vi "errorCheckArrayIndex.vi"(9 "<single path ele>":string, 10 "<req. obj>":string, 11 "Variant":variant) -> (3 "value":string)   [LabVIEW 2015, in "Zen Analytics.lvclass"]
uses:
  Zen Analytics.lvclass
  <vilib>/Utility/Data Type/Type Definitions/Data Type.ctl
  <vilib>/regexp/Match Regular Expression.xnode
  <vilib>/Utility/Data Type/NI_Data Type.lvlib
panel:
  out "error out":errorcluster
  in  "error in (no error)":errorcluster
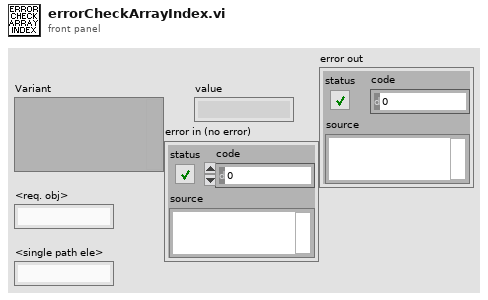
[diagram p1: front panel]
types:
  T1 = typedef "NI_Data Type.lvlib/Data Type.ctl" = enum8{"Invalid Type", "Void", "I8", "I16", "I32", "I64", "U8", "U16", "U32", "U64", "Single Float", "Double Float", "Extended Float", "Single Complex", "Double Complex", "Extended Complex", "Enum U8", "Enum U16", "Enum U32", "Enum U64", "Single Float With Unit", "Double Float With Unit", "Extended Float With Unit", "Single Complex with Unit", "Double Complex with Unit", "Extended Complex with Unit", "Boolean", "String", "Path", "Picture", "Tag", "Array", "Cluster", "Variant", "LV Variant", "Waveform", "Timestamp", "Digital Waveform", "Digital Data", "ExpressData", "Refnum", "External Data", "VI", "Poly VI", "LabVIEW Class Instance", "Fixed Point"}
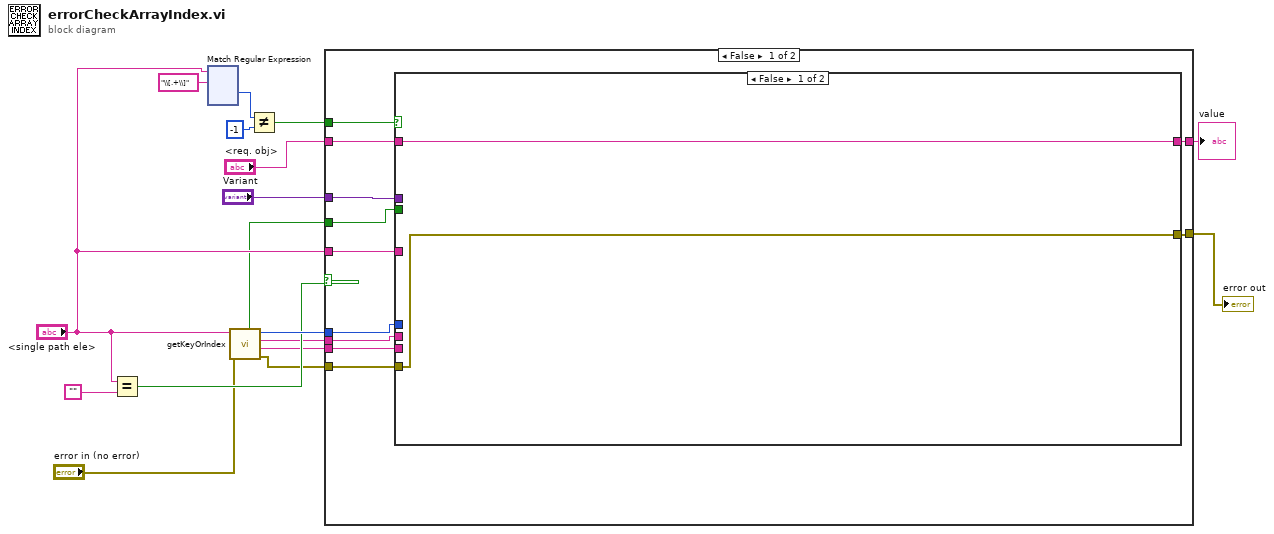
[diagram p0: block diagram]
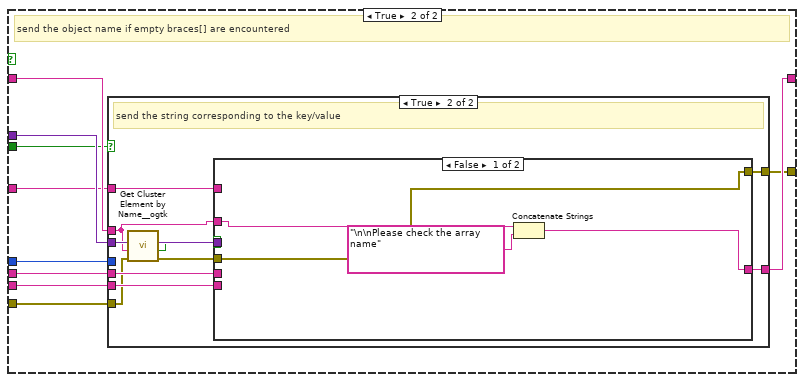
[diagram p2: hidden frame]
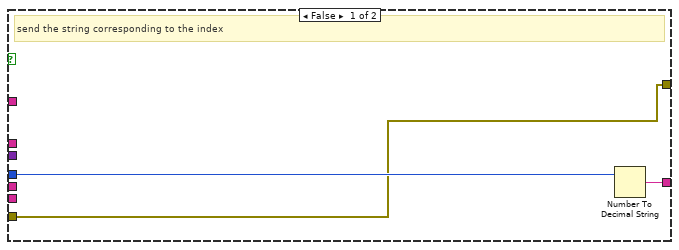
[diagram p3: hidden frame]
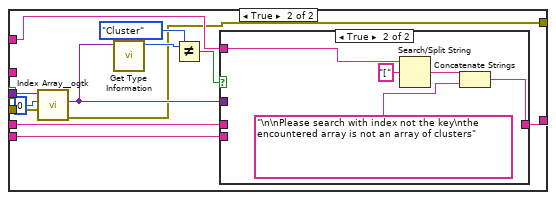
[diagram p4: hidden frame]
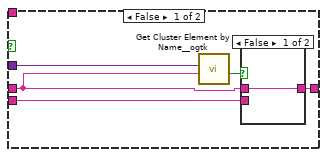
[diagram p5: hidden frame]
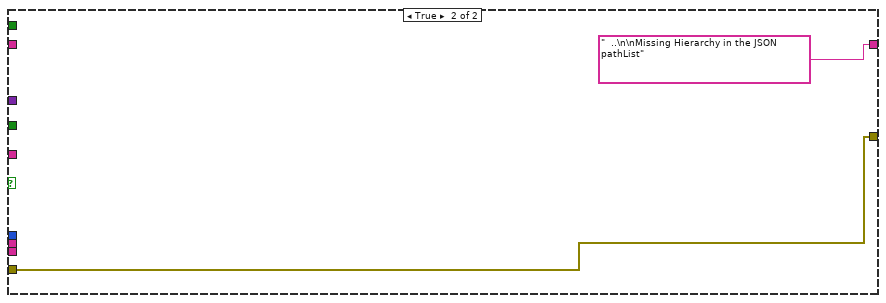
[diagram p7: hidden frame]
diagram:
  n1 = Equal?(x="<single path ele>", y="") -> (x = y?=w7:bool)
  n2 = xnode "Match Regular Expression"("input string"="<single path ele>", "regular expression"="\\[.+\\]") -> ("offset past match"=w10:i32)  [unwired: 4 in, 4 out]
  n3 = call "getKeyOrIndex.vi"("error in (no error)"="error in (no error)", "input string"="<single path ele>") -> ("error out"=w3:errorcluster, "value"=w4:string, "key"=w5:string, "index"=w16:i32, "keygiven?"=w6:bool)  [unwired: 5 in]
  n4 = Not Equal?(x=w10, y=-1) -> (x != y?=w12:bool)
  n5 = case shown="False" w7 {
    tunnel: "<req. obj>" -> [w28 _]
    tunnel: w4 -> [w27 _]
    tunnel: w16 -> [w26 _]
    tunnel: w6 -> [w25 _]
    tunnel: w5 -> [w24 _]
    tunnel: [w23 "  ..\n\nMissing Hierarchy in the JSON pathList" ("value")] -> w15
    tunnel: "Variant" -> [w22 _]
    tunnel: w12 -> [w21 _]
    tunnel: "<single path ele>" -> [w20 _]
    tunnel: w3 -> [w19 w83]
    tunnel: [w18 w83] -> w1
    frame False {
      n6 = case shown="False" w21 {
        tunnel: w28 -> [w30 w40]
        tunnel: w27 -> [_ w39]
        tunnel: w22 -> [_ w38]
        tunnel: w26 -> [_ w37]
        tunnel: w25 -> [_ w36]
        tunnel: w24 -> [_ w35]
        tunnel: [w30 w34] -> w23
        tunnel: w20 -> [_ w33]
        tunnel: w19 -> [w29 w32]
        tunnel: [w29 w31] -> w18
        frame False {
        }
        frame True {
          # "send the object name if empty braces[] are encountered"
          n7 = case shown="True" w36 {
            tunnel: w35 -> [_ w50]
            tunnel: [w42 w52] -> w34
            tunnel: w37 -> [w43 _]
            tunnel: w38 -> [_ w54]
            tunnel: w39 -> [_ w53]
            tunnel: w40 -> [_ w47]
            tunnel: w33 -> [_ w49]
            tunnel: w32 -> [w41 w46]
            tunnel: [w41 w44] -> w31
            frame False {
              # "send the string corresponding to the index"
              n8 = Number To Decimal String(number=w43) -> (decimal integer string=w42:string)  [unwired: 1 in]
            }
            frame True {
              # "send the string corresponding to the key/value"
              n9 = call <userlib>:"Get Cluster Element by Name__ogtk.vi"("error in (no error)"=w46, "Element Name"=w47, "Cluster"=w54) -> ("error out"=w45:errorcluster, "found?"=w48:bool, "VElement"=w51:variant)  [unwired: 6 in]
              n10 = case shown="False" w48 {
                tunnel: w53 -> [_ w70]
                tunnel: [w56 w69] -> w52
                tunnel: w51 -> [_ w68]
                tunnel: w50 -> [_ w66]
                tunnel: w49 -> [_ w61]
                tunnel: w47 -> [w58 _]
                tunnel: w45 -> [w55 w60]
                tunnel: [w55 w59] -> w44
                frame False {
                  n11 = Concatenate Strings(w58, "\n\nPlease check the array name" ("string")) -> (w56:string)
                }
                frame True {
                  n12 = call <userlib>:"Index Array__ogtk.vi"("error in (no error)"=w60, "Index (1D)"=u32 0, "MultiD Array"=w68) -> ("error out"=w59:errorcluster, "Array Element"=w65:variant)  [unwired: 7 in]
                  n13 = call <vilib>:"Get Type Information.vi"("Variant"=w65) -> ("Type"=w64:T1)  [unwired: 6 in, 4 out]
                  n14 = Not Equal?(x=w64, y=Data_Type."Cluster") -> (x != y?=w62:bool)
                  n15 = case shown="True" w62 {
                    tunnel: w70 -> [w75 _]
                    tunnel: [w74 w78] -> w69
                    tunnel: w66 -> [w73 _]
                    tunnel: w65 -> [w71 _]
                    tunnel: w61 -> [_ w81]
                    frame False {
                      n16 = call <userlib>:"Get Cluster Element by Name__ogtk.vi"("Element Name"=w73, "Cluster"=w71) -> ("found?"=w72:bool)  [unwired: 7 in, 2 out]
                      n17 = case shown="False" w72 {
                        tunnel: w75 -> [_ w77]
                        tunnel: [w76 w77] -> w74
                        tunnel: w73 -> [w76 _]
                        frame False {
                        }
                        frame True {
                        }
                      }
                    }
                    frame True {
                      n18 = Search/Split String(string=w81, search string/char (-)="[") -> (match + rest of string=w80:string)  [unwired: 1 in, 2 out]
                      n19 = Concatenate Strings(w80, "\n\nPlease search with index not the key\nthe encountered array is not an array of clusters" ("value")) -> (w78:string)
                    }
                  }
                }
              }
            }
          }
        }
      }
    }
    frame True {
    }
  }
  "value" <- w15
  "error out" <- w1
